vi "QUADRUPED TUNNING.vi"() -> ()   [LabVIEW 2017]
uses:
  <vilib>/Instr/_visa.llb/VISA Configure Serial Port (Instr).vi
panel:
  in  "Tab Control":enum32{"SETUP", "CALIBRATION"}(tab)
  out "VOLTAJE":dbl format="%_3g"
  in  "Search Button":bool
  in  "TEST":u16(ring) items=["CIF", "HIF", "CDF", "HDF", "CIA", "HIA", "CDA", "HDA"]
  in  "Save PinOut":bool
  in  "Download PinOut":bool
  in  "HDF PIN":dbl
  in  "Stop Button":bool
  in  "COM PORT":refnum<visa-resource-name>="COM3"
  in  "CDF PIN":dbl
  in  "HIF PIN":dbl
  in  "CIF PIN":dbl
  in  "HDA PIN":dbl
  in  "CDA PIN":dbl
  in  "HIA PIN":dbl
  in  "CIA PIN":dbl
  out "Numeric Indicator 2":dbl
  out "Numeric Indicator":dbl
  in  "Remove Button":bool
  in  "Add Button":bool
  in  "Knob":dbl(knob) scale=0.0..180.0
  # "INSTITUTO TECNOLOGICO DE CIUDAD GUZMAN"
  # "CUADRUPEDO PROJECT"
  # "Juan Jose Carranza Garcia"
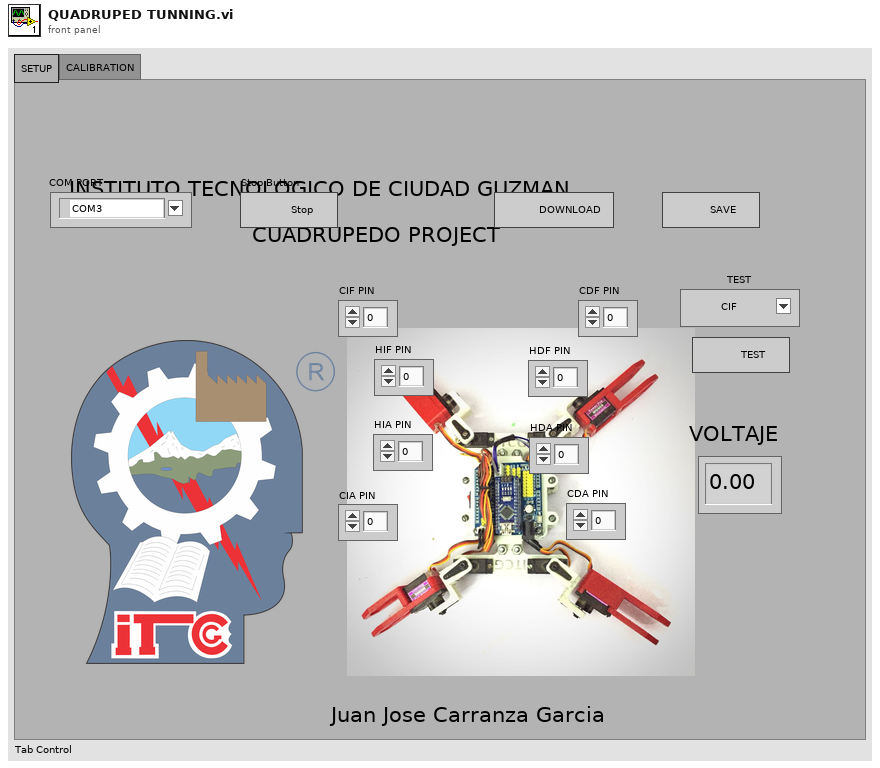
[diagram p1: front panel]
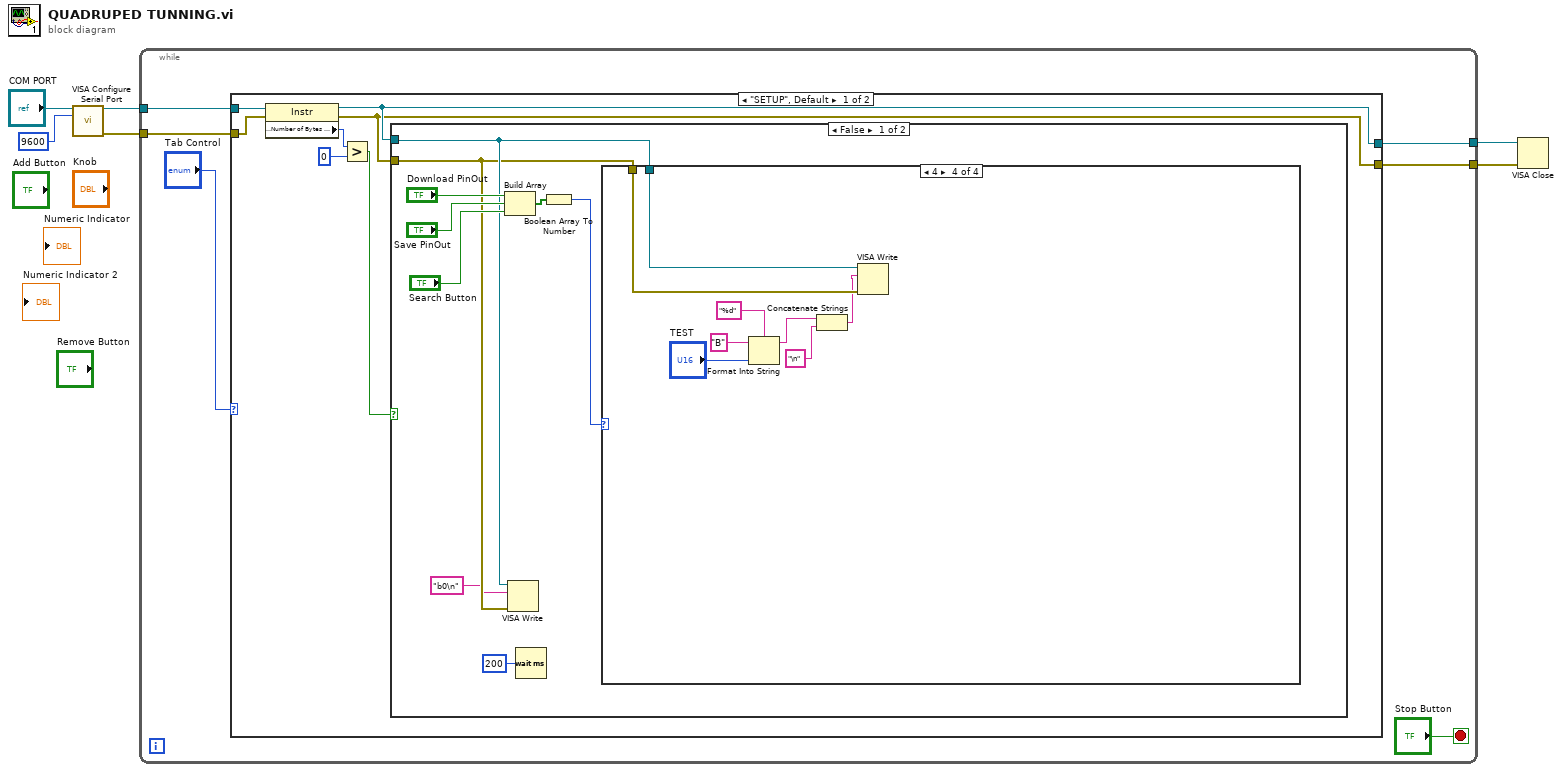
[diagram p0: block diagram]
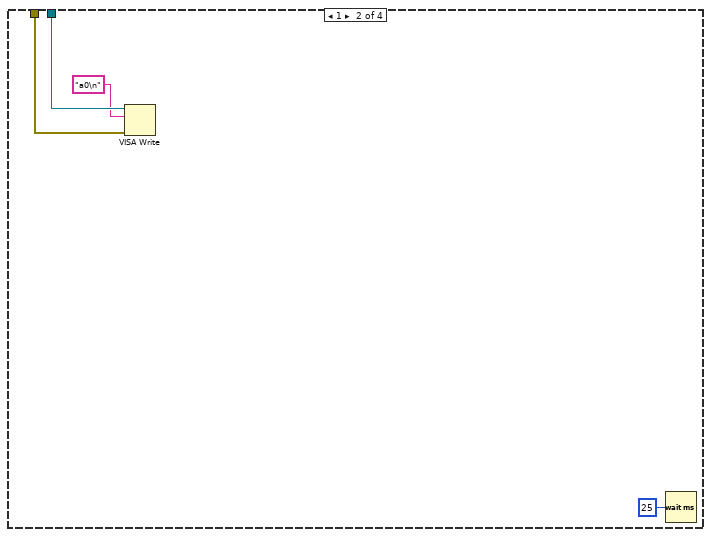
[diagram p3: hidden frame]
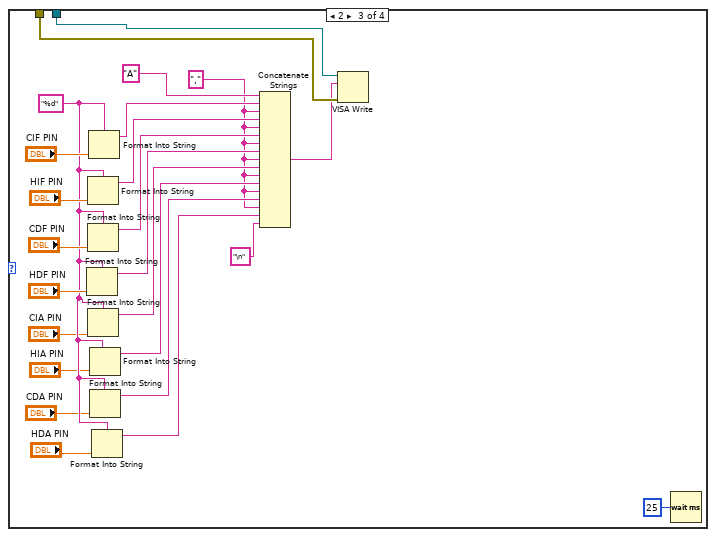
[diagram p4: hidden frame]
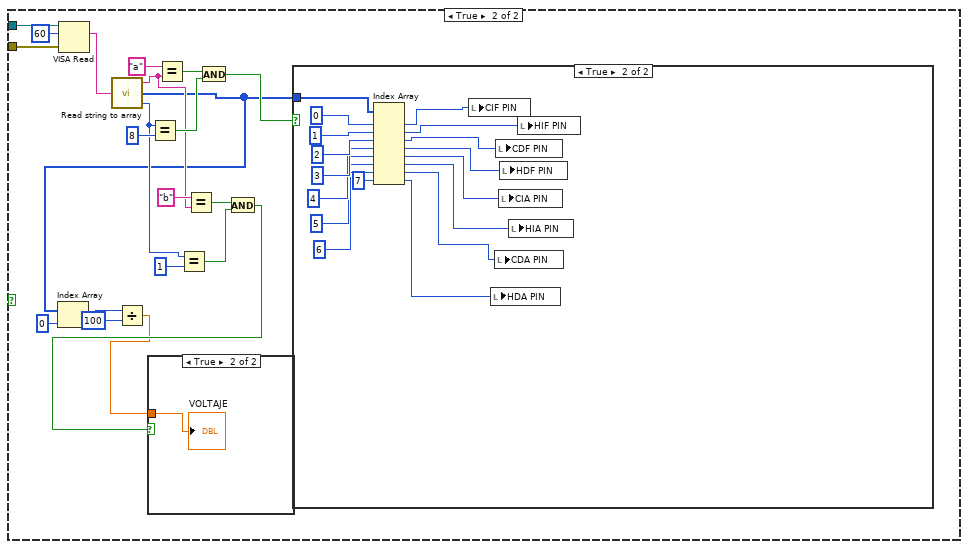
[diagram p5: hidden frame]
diagram:
  n1 = call-poly "VISA Configure Serial Port"("VISA resource name"="COM PORT", "baud rate (9600)"=u32 9600) -> ("VISA resource name out"=w4:refnum<visa-resource-name>, "error out"=w3:errorcluster)  [unwired: 12 in]
  n2 = while {
    tunnel: w4 -> [w10]
    tunnel: w3 -> [w9]
    tunnel: [w8] -> w2
    tunnel: [w7] -> w1
    stop <- "Stop Button" stop-if-true
    n3 = case shown="\"SETUP\", Default" "Tab Control" {
      tunnel: w10 -> [w17 w105]
      tunnel: w9 -> [w16 w104]
      tunnel: [w14 w105] -> w8
      tunnel: [w13 w104] -> w7
      frame "SETUP", Default {
        n4 = property class="Instr"(reference=w17, error in=w16) -> (reference out=w14:refnum<visa-resource-name>, error out=w13:errorcluster, "Serial Settings:Number of Bytes at Serial Port"=w19:u32)
        n5 = Greater?(x=w19, y=u32 0) -> (0:w15:bool)
        n6 = case shown="False" w15 {
          tunnel: w14 -> [w22 w85]
          tunnel: w13 -> [w21 w84]
          frame False {
            n7 = Build Array("Download PinOut", "Save PinOut", "Search Button") -> (w28:bool[])
            n8 = VISA Write(VISA resource name=w22, write buffer="b0\n", error in (no error)=w21) -> ()  [unwired: 3 out]
            n9 = Wait (ms)(milliseconds to wait=u32 200) -> ()  [unwired: 1 out]
            n10 = Boolean Array To Number(Boolean array=w28) -> (number=w25:u32)
            n11 = case shown="4" w25 {
              tunnel: w22 -> [_ w31 w46 w64]
              tunnel: w21 -> [_ w32 w45 w63]
              frame 0, Default {
              }
              frame 1 {
                n12 = VISA Write(VISA resource name=w31, write buffer="a0\n", error in (no error)=w32) -> ()  [unwired: 3 out]
                n13 = Wait (ms)(milliseconds to wait=u32 25) -> ()  [unwired: 1 out]
              }
              frame 2 {
                w33 = ","
                w51 = "%d" ("format string")
                n14 = Format Into String(format string=w51, "HDF PIN") -> (resulting string=w41:string)  [unwired: 2 in, 1 out]
                n15 = Format Into String(format string=w51, "HIF PIN") -> (resulting string=w43:string)  [unwired: 2 in, 1 out]
                n16 = Format Into String(format string=w51, "CDF PIN") -> (resulting string=w42:string)  [unwired: 2 in, 1 out]
                n17 = Format Into String(format string=w51, "CIA PIN") -> (resulting string=w40:string)  [unwired: 2 in, 1 out]
                n18 = Format Into String(format string=w51, "CIF PIN") -> (resulting string=w34:string)  [unwired: 2 in, 1 out]
                n19 = Format Into String(format string=w51, "HIA PIN") -> (resulting string=w39:string)  [unwired: 2 in, 1 out]
                n20 = Format Into String(format string=w51, "CDA PIN") -> (resulting string=w38:string)  [unwired: 2 in, 1 out]
                n21 = Format Into String(format string=w51, "HDA PIN") -> (resulting string=w37:string)  [unwired: 2 in, 1 out]
                n22 = Concatenate Strings("A" ("string"), w34, w33, w43, w33, w42, w33, w41, w33, w40, w33, w39, w33, w38, w33, w37, "\n" ("string")) -> (w44:string)
                n23 = VISA Write(VISA resource name=w46, write buffer=w44, error in (no error)=w45) -> ()  [unwired: 3 out]
                n24 = Wait (ms)(milliseconds to wait=u32 25) -> ()  [unwired: 1 out]
              }
              frame 4 {
                n25 = Format Into String(format string="%d", initial string="B", "TEST") -> (resulting string=w59:string)  [unwired: 1 in, 1 out]
                n26 = Concatenate Strings(w59, "\n" ("string")) -> (w57:string)
                n27 = VISA Write(VISA resource name=w64, write buffer=w57, error in (no error)=w63) -> ()  [unwired: 3 out]
              }
            }
          }
          frame True {
            n28 = VISA Read(VISA resource name=w85, byte count=u32 60, error in (no error)=w84) -> (read buffer=w82:string)  [unwired: 3 out]
            n29 = call "Read string to array.vi"("String"=w82) -> ("size(s)"=w71:i32, "Array"=w69:i32[], "caracter"=w72:string)  [unwired: 2 in]
            n30 = Index Array(array=w69, index=0) -> (element=w67:i32)
            n31 = Divide(x=w67, y=100) -> (x/y=w65:dbl)
            n32 = Equal?(x=w71, y=8) -> (x = y?=w78:bool)
            n33 = Equal?(x="a", y=w72) -> (x = y?=w79:bool)
            n34 = Equal?(x=w71, y=1) -> (x = y?=w73:bool)
            n35 = Equal?(x="b", y=w72) -> (x = y?=w74:bool)
            n36 = And(x=w79, y=w78) -> (x .and. y?=w77:bool)
            n37 = And(x=w74, y=w73) -> (x .and. y?=w70:bool)
            n38 = case shown="True" w70 {
              tunnel: w65 -> [_ w86]
              frame False {
              }
              frame True {
                "VOLTAJE" <- w86
              }
            }
            n39 = case shown="True" w77 {
              tunnel: w69 -> [_ w102]
              frame False {
              }
              frame True {
                n40 = Index Array(array=w102, index #1=0 ("index"), index #2=1 ("index"), index #3=2 ("index"), index #4=3 ("index"), index #5=4 ("index"), index #6=5 ("index"), index #7=6 ("index"), index #8=7 ("index")) -> (element #1=w103:i32, element #2=w93:i32, element #3=w92:i32, element #4=w91:i32, element #5=w90:i32, element #6=w89:i32, element #7=w88:i32, element #8=w87:i32)
                n41 = local write "CIF PIN"(w103) -> ()
                n42 = local write "HDA PIN"(w87) -> ()
                n43 = local write "CDA PIN"(w88) -> ()
                n44 = local write "CDF PIN"(w92) -> ()
                n45 = local write "CIA PIN"(w90) -> ()
                n46 = local write "HDF PIN"(w91) -> ()
                n47 = local write "HIA PIN"(w89) -> ()
                n48 = local write "HIF PIN"(w93) -> ()
              }
            }
          }
        }
      }
      frame "CALIBRATION" {
      }
    }
  }
  n49 = VISA Close(VISA resource name=w2, error in (no error)=w1) -> ()  [unwired: 1 out]
